vi "Day 1 task 1.vi"() -> ()   [LabVIEW 2022 SP3]
uses:
  <vilib>/regexp/Match Regular Expression.xnode
panel:
  out "sum":i32
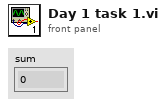
[diagram p1: front panel]
diagram:
  (unwired) "1abc2\npqr3stu8vwx\na1b2c3d4e5f\ntreb7uchet"
  n1 = Spreadsheet String To Array(delimiter (Tab)="\n", format string="%s", spreadsheet string="cmpptgjc3qhcjxcbcqgqkxhrms\n9sixonefour\neighttwo2twofour9\n7eightseveneightthree\ntlnllks2jcfdlgsjbhpfnineone\none44fivesevenjzsfzddg\n787seveneight75five\n7q7nine3\nhlqphphn5dtzzbqvk3three8seven\nninekkbvsfq8seven7321bpdcdh\n9kxgfxntgdzs1ns5\nnineblxtnrt79t8fourbcqdzpb\n3mjqgthreeseven36gkvvvqppx\nzpcvkjjqeight94one82mrvfzdvlgjgkhj\nnine11\nrnscpccv8\n7eightrcqnbtkn\nfour31zqgrccc4eight\ntwo65fourfourt1\ntwomg2764threesix\n546grjcrsix9\n4ffourfourff1\ndpfkcrzjxr8four\n641one\nkseven8\ntwo4four\nldzpzgch325hsttqvmp9foureightmvsknbd\nonexrbclqlnvp5kqtrsgdh8nine\nrk9qfzvszksjqsixg\ndcnhlcqzhthreebhrnfgjbfive1threetwo53\n1tw...", array type (2D Dbl)=string[] []) -> (array=w3:string[])
  n2 = for {
    tunnel: w3 -> [w15] mode=indexing
    tunnel: [w8] -> w2 mode=indexing
    n3 = Reverse String(1:w15) -> (0:w10:string)
    n4 = xnode "Match Regular Expression"("input string"=w10, "regular expression"="\\d") -> ("whole match"=w11:string, "error out"=w16:errorcluster)  [unwired: 4 in, 3 out]
    n5 = xnode "Match Regular Expression"("input string"=w15, "regular expression"="\\d", "error in"=w16) -> ("whole match"=w12:string)  [unwired: 3 in, 4 out]
    n6 = Concatenate Strings(w12, w11) -> (w9:string)
    n7 = Decimal String To Number(string=w9) -> (number=w8:i32)  [unwired: 2 in, 1 out]
  }
  n8 = Add Array Elements(numeric array=w2) -> (sum=→"sum":i32)
